vi "gmmregRegistrationTest.vi"() -> ()   [LabVIEW 2017]
panel:
  out "out":dbl[][](array[numeric])
  in  "Array":dbl[][](array[numeric])=[[255.0, 255.0, 0.0]]
  out "params out":dbl[][](array[numeric]) format="%#_6e"
  out "XY Graph":cluster{dbl[], dbl[]}[](graph)
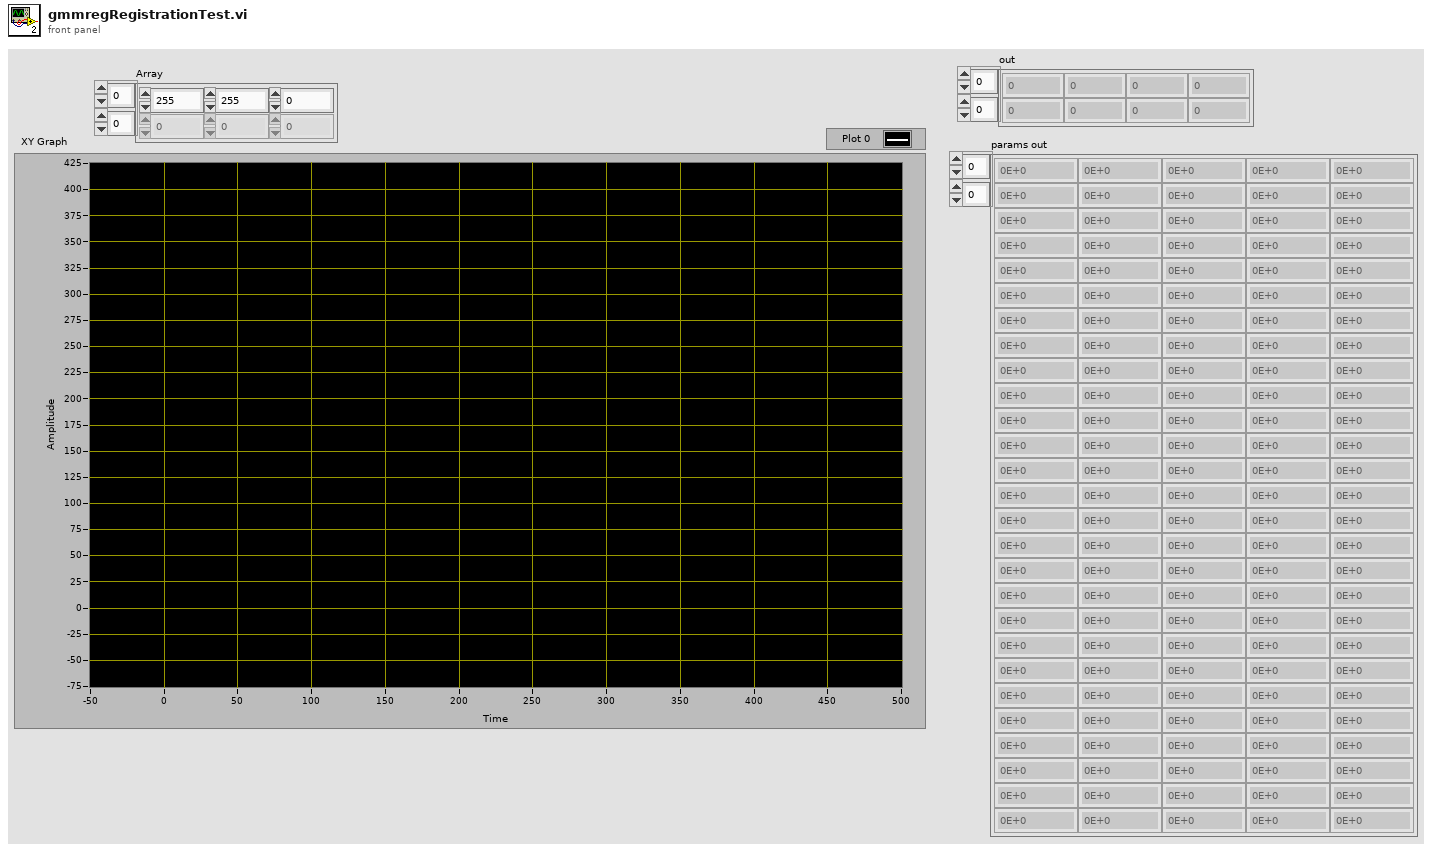
[diagram p1: front panel]
types:
  T1 = cluster{"imaging (model)":dbl[], "imaging (model)":dbl[]}
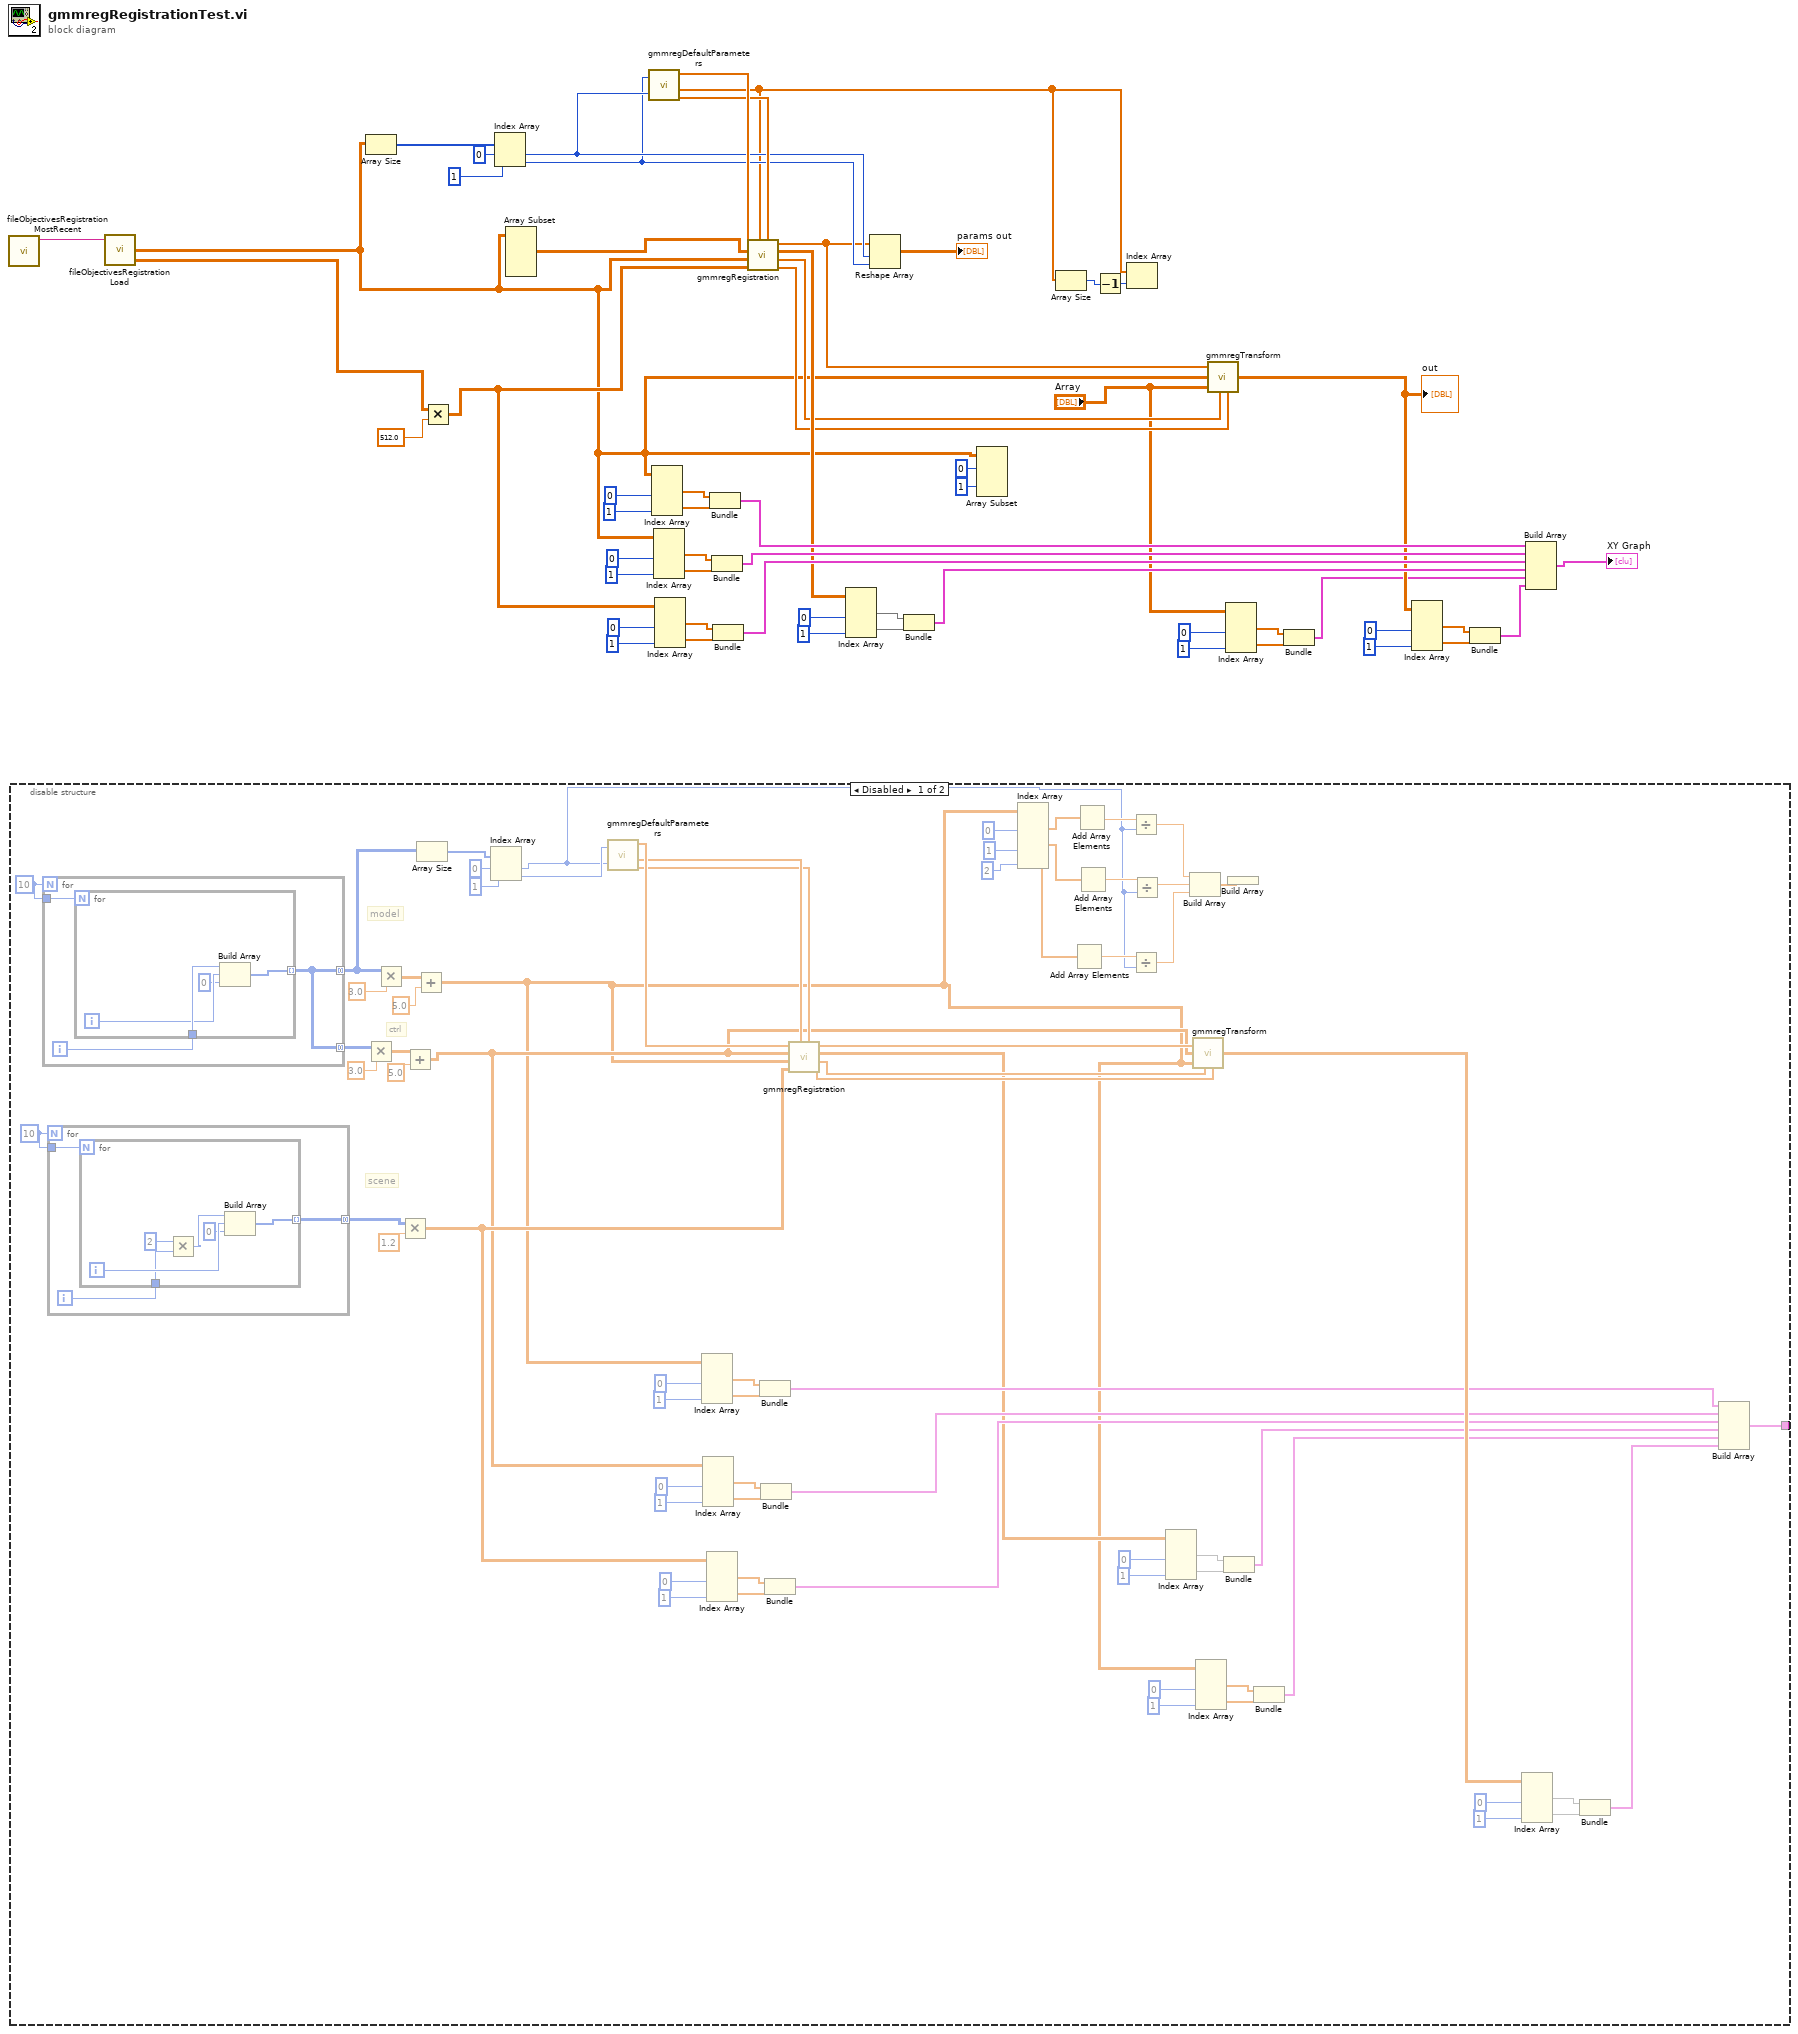
[diagram p0: block diagram]
diagram:
  n1 = call "fileObjectivesRegistrationMostRecent.vi"() -> ("f"=w3:string)  [unwired: 1 in]
  n2 = disable-structure shown="Disabled" {
    disable-tunnel: [w81 _] -> _
    frame Disabled {
      w127 = 10
      w128 = 10
      # "ctrl"
      # "scene"
      # "model"
      n3 = for {
        N: w128 -> [_]
        tunnel: w128 -> [w140]
        tunnel: [w138] -> w115 mode=concatenating
        tunnel: [w138] -> w120 mode=concatenating
        i -> [w139]
        n4 = for {
          N: w140 -> [_]
          tunnel: w139 -> [w144]
          tunnel: [w142] -> w138 mode=indexing
          i -> [w143]
          n5 = Build Array(w144, w143, 0 ("element")) -> (w142:i32[])
        }
      }
      n6 = for {
        N: w127 -> [_]
        tunnel: w127 -> [w131]
        tunnel: [w129] -> w126 mode=concatenating
        i -> [w130]
        n7 = for {
          N: w131 -> [_]
          tunnel: w130 -> [w134]
          tunnel: [w136] -> w129 mode=indexing
          i -> [w137]
          n8 = Multiply(x=2, y=w134) -> (x*y=w132:i32)
          n9 = Build Array(w132, w137, 0 ("element")) -> (w136:i32[])
        }
      }
      n10 = Multiply(x=w120, y=3.0) -> (x*y=w119:dbl[][])
      n11 = Multiply(x=w115, y=3.0) -> (x*y=w123:dbl[][])
      n12 = Multiply(x=w126, y=1.2) -> (x*y=w98:dbl[][])
      n13 = Add(x=w119, y=5.0) -> (x+y=w94:dbl[][])
      n14 = Add(x=w123, y=5.0) -> (x+y=w57:dbl[][])
      n15 = Array Size(array=w115) -> (size(s)=w113:i32[])
      n16 = Index Array(array=w113, index #1=0 ("index"), index #2=1 ("index")) -> (element #1=w67:i32, element #2=w72:i32)
      n17 = call "gmmregDefaultParameters.vi"("D (3)"=w72, "nctrlPts"=w67) -> ("param0"=w114:dbl[], "default scales"=w112:dbl[], "deault lambdas"=w111:dbl[])  [unwired: 1 out]
      n18 = Index Array(array=w57, index (col) #1=0 ("index"), index (col) #2=1 ("length")) -> (element #1=w109:dbl[], element #2=w110:dbl[])  [unwired: 2 in]
      n19 = Index Array(array=w94, index (col) #1=0 ("index"), index (col) #2=1 ("length")) -> (element #1=w104:dbl[], element #2=w103:dbl[])  [unwired: 2 in]
      n20 = Index Array(array=w98, index (col) #1=0 ("index"), index (col) #2=1 ("length")) -> (element #1=w101:dbl[], element #2=w102:dbl[])  [unwired: 2 in]
      n21 = Bundle(w109, w110) -> (w84:cluster{dbl[], dbl[]})  [unwired: 1 in]
      n22 = Bundle(w104, w103) -> (w83:cluster{dbl[], dbl[]})  [unwired: 1 in]
      n23 = Bundle(w101, w102) -> (w82:cluster{dbl[], dbl[]})  [unwired: 1 in]
      n24 = call "gmmregRegistration.vi"("lambda"=w111, "scale"=w112, "scene"=w98, "model"=w57, "ctrlPoints"=w94, "param0"=w114) -> ("denormParams out"=w95:dbl[], "normParams out"=w96:dbl[], "out"=w74:dbl[][], "param0 out"=w97:dbl[])  [unwired: 2 in]
      n25 = Index Array(array=w57, index (col) #1=0 ("index"), index (col) #2=1 ("index"), index (col) #3=2 ("index")) -> (element #1=w60:dbl[], element #2=w59:dbl[], element #3=w58:dbl[])  [unwired: 3 in]
      n26 = Add Array Elements(numeric array=w58) -> (sum=w68:dbl)
      n27 = Add Array Elements(numeric array=w60) -> (sum=w70:dbl)
      n28 = Add Array Elements(numeric array=w59) -> (sum=w69:dbl)
      n29 = Divide(x=w70, y=w67) -> (x/y=w64:dbl)
      n30 = Divide(x=w68, y=w67) -> (x/y=w66:dbl)
      n31 = Divide(x=w69, y=w67) -> (x/y=w65:dbl)
      n32 = Index Array(array=w74, index (col) #1=0 ("index"), index (col) #2=1 ("length")) -> (element #1=w77:dbl[], element #2=w78:dbl[])  [unwired: 2 in]
      n33 = Build Array(w64, w65, w66) -> (w71:dbl[])
      n34 = call "gmmregTransform.vi"("param0"=w97, "ctrlPts"=w94, "pts"=w57, "normParams"=w96, "denormParams"=w95) -> ("out"=w85:dbl[][])  [unwired: 4 in]
      n35 = Index Array(array=w57, index (col) #1=0 ("index"), index (col) #2=1 ("length")) -> (element #1=w91:dbl[], element #2=w90:dbl[])  [unwired: 2 in]
      n36 = Bundle("out"=w77, "out"=w78) -> (w73:cluster{"out":dbl[], "out":dbl[]})  [unwired: 1 in]
      n37 = Build Array(w71) -> ()  [unwired: 1 out]
      n38 = Bundle(w91, w90) -> (w79:cluster{dbl[], dbl[]})  [unwired: 1 in]
      n39 = Index Array(array=w85, index (col) #1=0 ("index"), index (col) #2=1 ("length")) -> (element #1=w88:dbl[], element #2=w89:dbl[])  [unwired: 2 in]
      n40 = Bundle("out"=w88, "out"=w89) -> (w80:cluster{"out":dbl[], "out":dbl[]})  [unwired: 1 in]
      n41 = Build Array(w84, w83, w82, w73, w79, w80) -> (w81:cluster{"out":dbl[], "out":dbl[]}[])
    }
    frame Enabled {
    }
  }
  n42 = call "fileObjectivesRegistrationLoad.vi"("objectiveRegistrationFilePath"=w3) -> ("imaging (model)"=w2:dbl[][], "optogenetics (scene)"=w1:dbl[][])  [unwired: 4 in, 3 out]
  n43 = Array Size(array=w2) -> (size(s)=w45:i32[])
  n44 = Multiply(x=w1, y=512.0) -> (x*y=w42:dbl[][])
  n45 = Index Array(array=w45, index #1=0 ("index"), index #2=1 ("index")) -> (element #1=w41:i32, element #2=w40:i32)
  n46 = Array Subset(array=w2) -> (w4:dbl[][])  [unwired: 4 in]
  n47 = call "gmmregDefaultParameters.vi"("D (3)"=w40, "nctrlPts"=w41) -> ("param0"=w56:dbl[], "default scales"=w37:dbl[], "deault lambdas"=w55:dbl[])  [unwired: 1 out]
  n48 = Index Array(array=w2, index (col) #1=0 ("index"), index (col) #2=1 ("length")) -> (element #1=w12:dbl[], element #2=w11:dbl[])  [unwired: 2 in]
  n49 = Index Array(array=w2, index (col) #1=0 ("index"), index (col) #2=1 ("length")) -> (element #1=w17:dbl[], element #2=w18:dbl[])  [unwired: 2 in]
  n50 = Index Array(array=w42, index (col) #1=0 ("index"), index (col) #2=1 ("length")) -> (element #1=w20:dbl[], element #2=w19:dbl[])  [unwired: 2 in]
  n51 = Bundle("imaging (model)"=w12, "imaging (model)"=w11) -> (w54:T1)  [unwired: 1 in]
  n52 = Bundle("imaging (model)"=w17, "imaging (model)"=w18) -> (w53:T1)  [unwired: 1 in]
  n53 = Bundle(w20, w19) -> (w52:cluster{dbl[], dbl[]})  [unwired: 1 in]
  n54 = call "gmmregRegistration.vi"("lambda"=w55, "scale"=w37, "scene"=w42, "model"=w2, "ctrlPoints"=w4, "param0"=w56) -> ("denormParams out"=w7:dbl[], "normParams out"=w8:dbl[], "out"=w23:dbl[][], "param0 out"=w38:dbl[])  [unwired: 2 in]
  n55 = Index Array(array=w23, index (col) #1=0 ("index"), index (col) #2=1 ("length")) -> (element #1=w50:dbl[], element #2=w51:dbl[])  [unwired: 2 in]
  n56 = Reshape Array(w38, w41, w40) -> (→"params out":dbl[][])
  n57 = Bundle("out"=w50, "out"=w51) -> (w47:cluster{"out":dbl[], "out":dbl[]})  [unwired: 1 in]
  n58 = Array Subset(array=w2, index (row)=0 ("index"), length (row)=1 ("length")) -> ()  [unwired: 2 in, 1 out]
  n59 = Array Size(array=w37) -> (size(s)=w36:i32)
  n60 = Decrement(x=w36) -> (x-1=w35:i32)
  n61 = Index Array(array=w37, index=w35) -> ()  [unwired: 1 out]
  n62 = call "gmmregTransform.vi"("param0"=w38, "ctrlPts"=w2, "pts"="Array", "normParams"=w8, "denormParams"=w7) -> ("out"=w30:dbl[][])  [unwired: 4 in]
  "out" <- w30
  n63 = Index Array(array="Array", index (col) #1=0 ("index"), index (col) #2=1 ("length")) -> (element #1=w27:dbl[], element #2=w28:dbl[])  [unwired: 2 in]
  n64 = Bundle("Array"=w27, "Array"=w28) -> (w24:cluster{"Array":dbl[], "Array":dbl[]})  [unwired: 1 in]
  n65 = Index Array(array=w30, index (col) #1=0 ("index"), index (col) #2=1 ("length")) -> (element #1=w32:dbl[], element #2=w31:dbl[])  [unwired: 2 in]
  n66 = Bundle("out"=w32, "out"=w31) -> (w29:cluster{"out":dbl[], "out":dbl[]})  [unwired: 1 in]
  n67 = Build Array(w54, w53, w52, w47, w24, w29) -> (→"XY Graph":cluster{"out":dbl[], "out":dbl[]}[])
